vi "axex_read_cells_vector.vi"(6 "vertical vector (False)":bool, 7 "error proof read (True)":bool=TRUE, 8 "error in":errorcluster, 9 "vector size":i32=1 min=1, 10 "top-left cell":T1, 11 "AX Excel instance in":T2) -> (0 "error out":errorcluster, 2 "strings vector":string[](array[string]), 3 "AX Excel instance out":T2)   [LabVIEW 2020, in "AX Excel.lvlib"]
doc: "Call this to read vector of cells. The vector starts at given coordinates and has 'vector size' cells. The coordinates of top-left cell may be given as [column,row] index or cell name such as A1, AB66, ... with priority of cell name.\n\n'Error proof read' option means the VI will first try to read entire array at once as usually. If it fails it probably means some cell has invalid content so it will try to read the cells one by one so it should always return the array (with empty cells for the invalid cells). But keep in mind this can be painfully slow for larger arrays."
uses:
  AX Excel.lvlib
  axex_instance.ctl
  axex_cell_xy.ctl
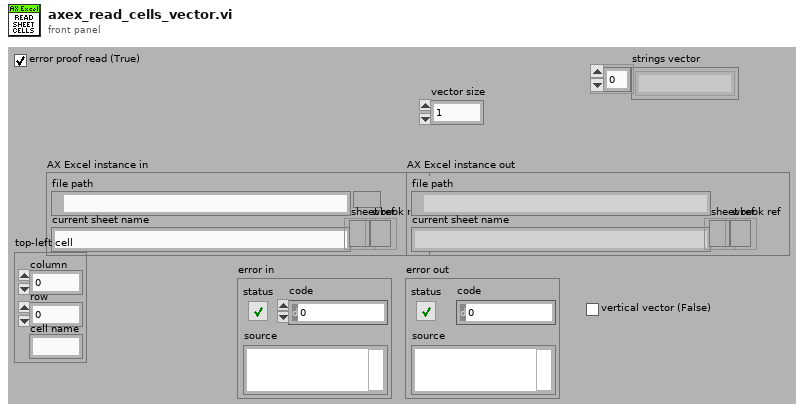
[diagram p1: front panel]
types:
  T1 = typedef "AX Excel.lvlib/axex_cell_xy.ctl" = cluster{"column":i32, "row":i32, "cell name":string}
  T2 = typedef "AX Excel.lvlib/axex_instance.ctl" = cluster{"file path":path, "current sheet name":string, "sheet ref":refnum<k7>, "wbook ref":refnum<k7>}
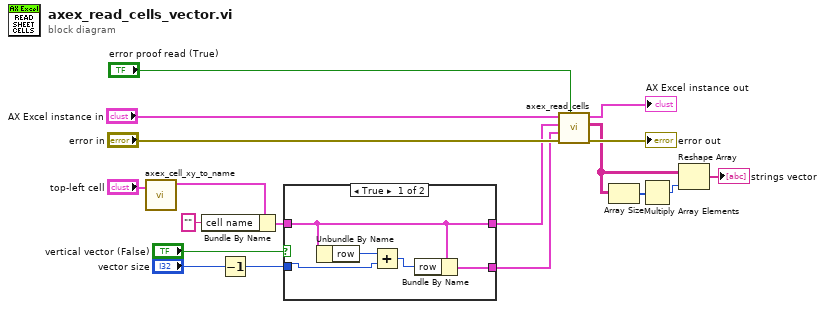
[diagram p0: block diagram]
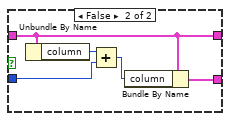
[diagram p2: hidden frame]
diagram:
  n1 = call "axex_cell_xy_to_name.vi"("cell xy in"="top-left cell") -> ("cell xy out"=w11:T1)  [unwired: 1 in, 3 out]
  n2 = Bundle By Name(cluster=w11, "cell name"="") -> (w9:T1)
  n3 = Decrement(x="vector size") -> (x-1=w7:i32)
  n4 = case shown="True" "vertical vector (False)" {
    tunnel: w9 -> [w22 w27]
    tunnel: w7 -> [w19 w25]
    tunnel: [w22 w27] -> w6
    tunnel: [w23 w28] -> w5
    frame True {
      n5 = Unbundle By Name(w22) -> ("row"=w21:i32)
      n6 = Add(x=w21, y=w19) -> (x+y=w20:i32)
      n7 = Bundle By Name(cluster=w22, "row"=w20) -> (w23:T1)
    }
    frame False {
      n8 = Unbundle By Name(w27) -> ("column"=w26:i32)
      n9 = Add(x=w26, y=w25) -> (x+y=w24:i32)
      n10 = Bundle By Name(cluster=w27, "column"=w24) -> (w28:T1)
    }
  }
  n11 = call "axex_read_cells.vi"("error proof read (True)"="error proof read (True)", "error in"="error in", "right bottom cell"=w5, "top left cell"=w6, "AX Excel instance in"="AX Excel instance in") -> ("error out"=→"error out":errorcluster, "cell array"=w4:string[][], "AX Excel instance out"=→"AX Excel instance out":T2)  [unwired: 3 in, 1 out]
  n12 = Array Size(array=w4) -> (size(s)=w3:i32[])
  n13 = Multiply Array Elements(1:w3) -> (0:w2:i32)
  n14 = Reshape Array(w4, w2) -> (→"strings vector":string[])
